vi "Write (SubVI).vi"(8 "error in":errorcluster, 10 "Запрос":string, 11 "Param in":T1={"ReadIntParam"=TRUE, "ReadDescrParam"=FALSE, "ReadFloatParam"=TRUE, "debug"=FALSE, "ReadJSON"=TRUE, "IP_address"="192.168.1.216", "N_attempts"=3, "type_con"=enum."TCP", "MB_address"=1, "VISA"="COM1", "connection ID"=refnum, "nameDevices"="", "timeout"=0, "port"=0, "type_version"="0F0C0001", "baud_rate"=115200, "VersionControl"=TRUE, "TCP_conn"=TRUE, "WindowSize"=700}) -> (0 "error out":errorcluster, 3 "Param out":T1={"ReadIntParam"=TRUE, "ReadDescrParam"=FALSE, "ReadFloatParam"=TRUE, "debug"=FALSE, "ReadJSON"=TRUE, "IP_address"="192.168.1.216", "N_attempts"=3, "type_con"=enum."TCP", "MB_address"=1, "VISA"="COM1", "connection ID"=refnum, "nameDevices"="", "timeout"=0, "port"=0, "type_version"="0F0C0001", "baud_rate"=115200, "VersionControl"=TRUE, "TCP_conn"=TRUE, "WindowSize"=700})   [LabVIEW 2017, in "LV_Unicorn.lvlib"]
uses:
  LV_Unicorn.lvlib
  Control/unicorn_conn.ctl
panel:
  out "bytes written":i32
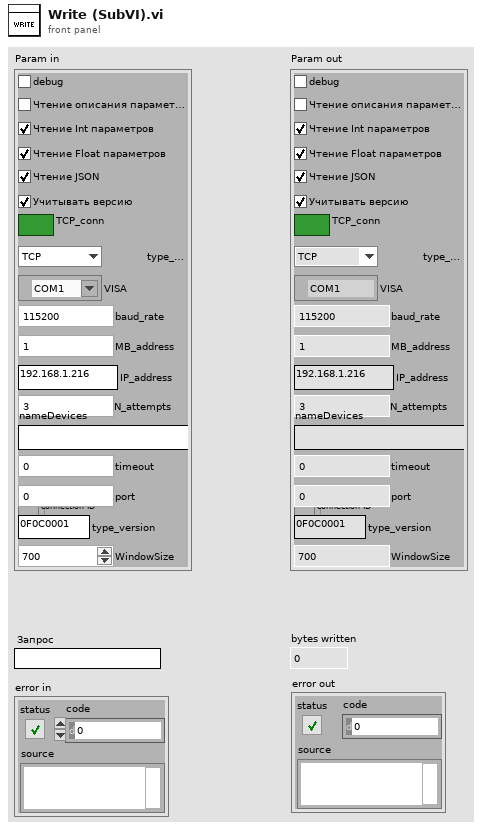
[diagram p1: front panel]
types:
  T1 = typedef "LV_Unicorn.lvlib/unicorn_conn.ctl" = cluster{"ReadIntParam":bool, "ReadDescrParam":bool, "ReadFloatParam":bool, "debug":bool, "ReadJSON":bool, "IP_address":string, "N_attempts":i32, "type_con":enum16{"Serial", "TCP"}, "MB_address":i32, "VISA":refnum<visa-resource-name>, "connection ID":refnum<k5>, "nameDevices":string, "timeout":i32, "port":u16, "type_version":string, "baud_rate":u32, "VersionControl":bool, "TCP_conn":bool, "WindowSize":i32}
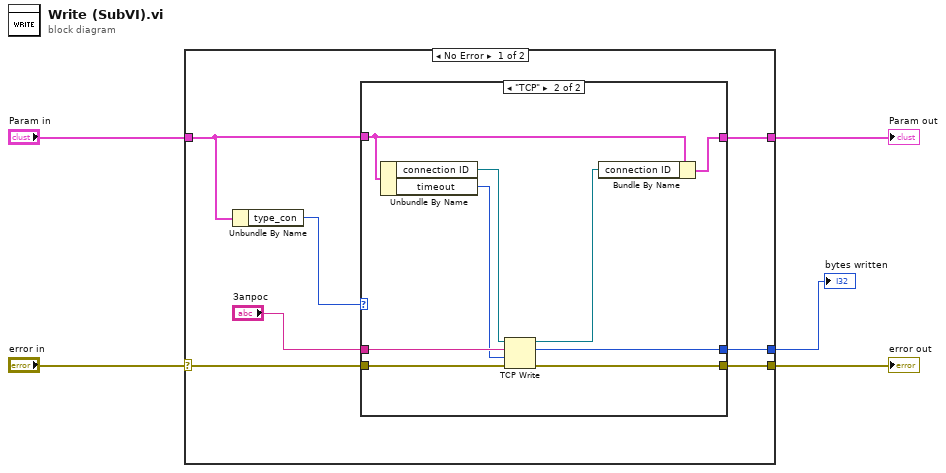
[diagram p0: block diagram]
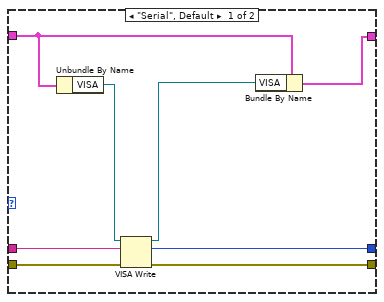
[diagram p2: hidden frame]
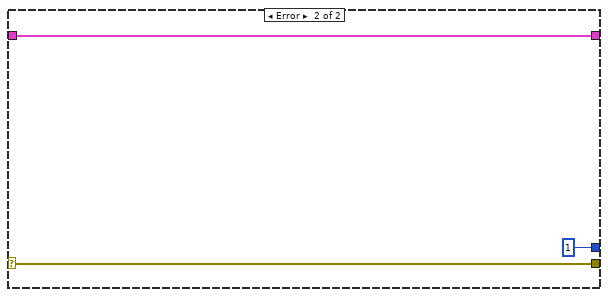
[diagram p3: hidden frame]
diagram:
  n1 = case shown="No Error" "error in" {
    selector: "error in" -> [w9 w32]
    tunnel: [w11 w32] -> w5
    tunnel: "Param in" -> [w8 w31]
    tunnel: [w7 w31] -> w3
    tunnel: [w6 u32 1 ("return count")] -> w1
    frame No Error {
      n2 = Unbundle By Name(w8) -> ("type_con"=w12:enum16{"Serial", "TCP"})
      n3 = case shown="\"TCP\"" w12 {
        tunnel: "Запрос" -> [w20 w29]
        tunnel: [w19 w28] -> w11
        tunnel: w9 -> [w18 w27]
        tunnel: w8 -> [w16 w24]
        tunnel: [w14 w22] -> w7
        tunnel: [w13 w21] -> w6
        frame "Serial", Default {
          n4 = Unbundle By Name(w16) -> ("VISA"=w17:refnum<visa-resource-name>)
          n5 = VISA Write(VISA resource name=w17, write buffer=w20, error in (no error)=w18) -> (VISA resource name out=w15:refnum<visa-resource-name>, return count=w13:u32, error out=w19:errorcluster)
          n6 = Bundle By Name(cluster=w16, "VISA"=w15) -> (w14:T1)
        }
        frame "TCP" {
          n7 = Unbundle By Name(w24) -> ("connection ID"=w26:refnum<k5>, "timeout"=w25:i32)
          n8 = TCP Write(connection ID=w26, data in=w29, error in (no error)=w27, 9:w25) -> (connection ID out=w23:refnum<k5>, bytes written=w21:i32, error out=w28:errorcluster)
          n9 = Bundle By Name(cluster=w24, "connection ID"=w23) -> (w22:T1)
        }
      }
    }
    frame Error {
    }
  }
  "error out" <- w5
  "Param out" <- w3
  "bytes written" <- w1
